vi "CMD_PRINT_TEST.vi"() -> ()   [LabVIEW 2017]
panel:
  in  "error in (no error)":errorcluster
  out "error out":errorcluster
  out "standard output":string
  in  "command line":string="cmd /c COPY /B \"\\\"D:\\AA TODAYS\\MAGNETIC\\MAGNETIC SOFT\\MagneticAssymbly\\data\\RATING_PRINT.prn\\\"\" \"\\\"\\\\DESKTOP-ICM4L4Q\\ZDesigner ZD421_MAGNECTIC\\\"\"\n"
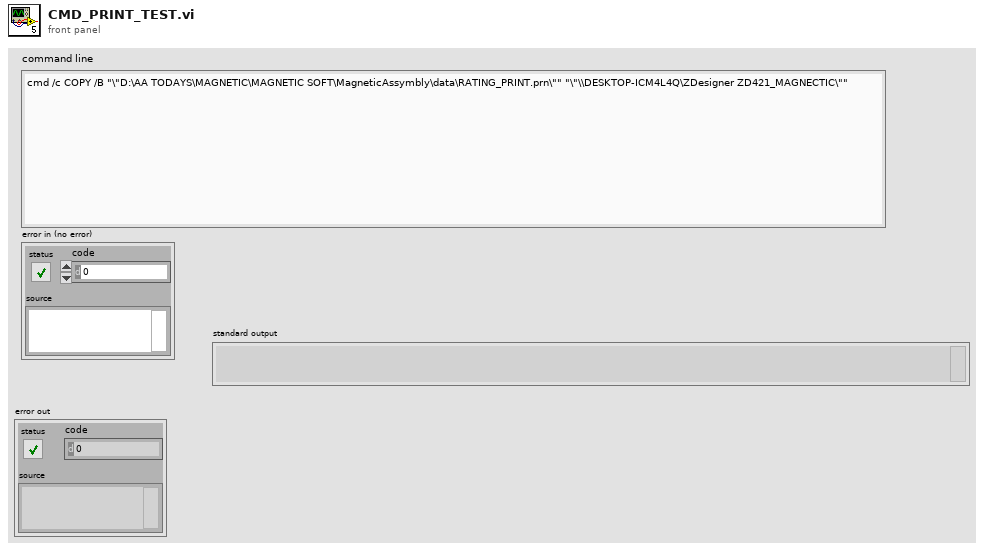
[diagram p1: front panel]
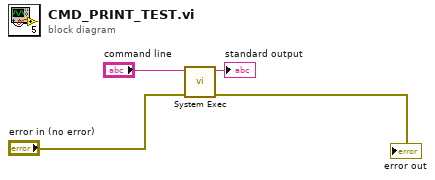
[diagram p0: block diagram]
diagram:
  n1 = call <vilib>:"System Exec.vi"("error in (no error)"="error in (no error)", "command line"="command line") -> ("error out"=→"error out":errorcluster, "standard output"=→"standard output":string)  [unwired: 6 in, 2 out]
